vi "TagContainer-UpdateUI.vi"(7 "VIRef(Caller VI)":refnum<vi>, 8 "error in (no error)":errorcluster, 9 "force update(F)":bool, 11 "TagContainer":T1) -> (0 "error out":errorcluster, 3 "TagContainer(dup)":T1)   [LabVIEW 2017, in "TagContainer.lvlib"]
uses:
  TagContainer.lvlib
  Program Files (x86)/National Instruments/LabVIEW 2020/user.lib/_OpenG.lib/array/array.llb/Index 1D Array Elements (Variant)__ogtk.vi
  Typedef/TagContainer.ctl
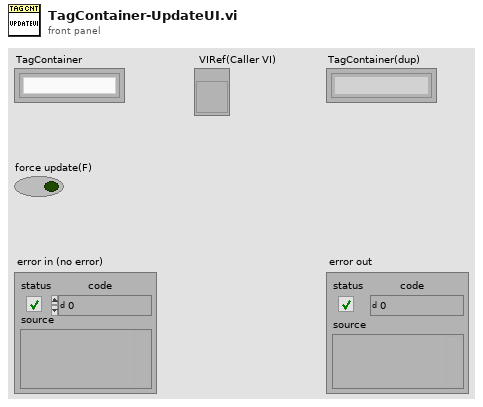
[diagram p1: front panel]
types:
  T1 = typedef "TagContainer.lvlib/TagContainer.ctl" = refnum<k1>
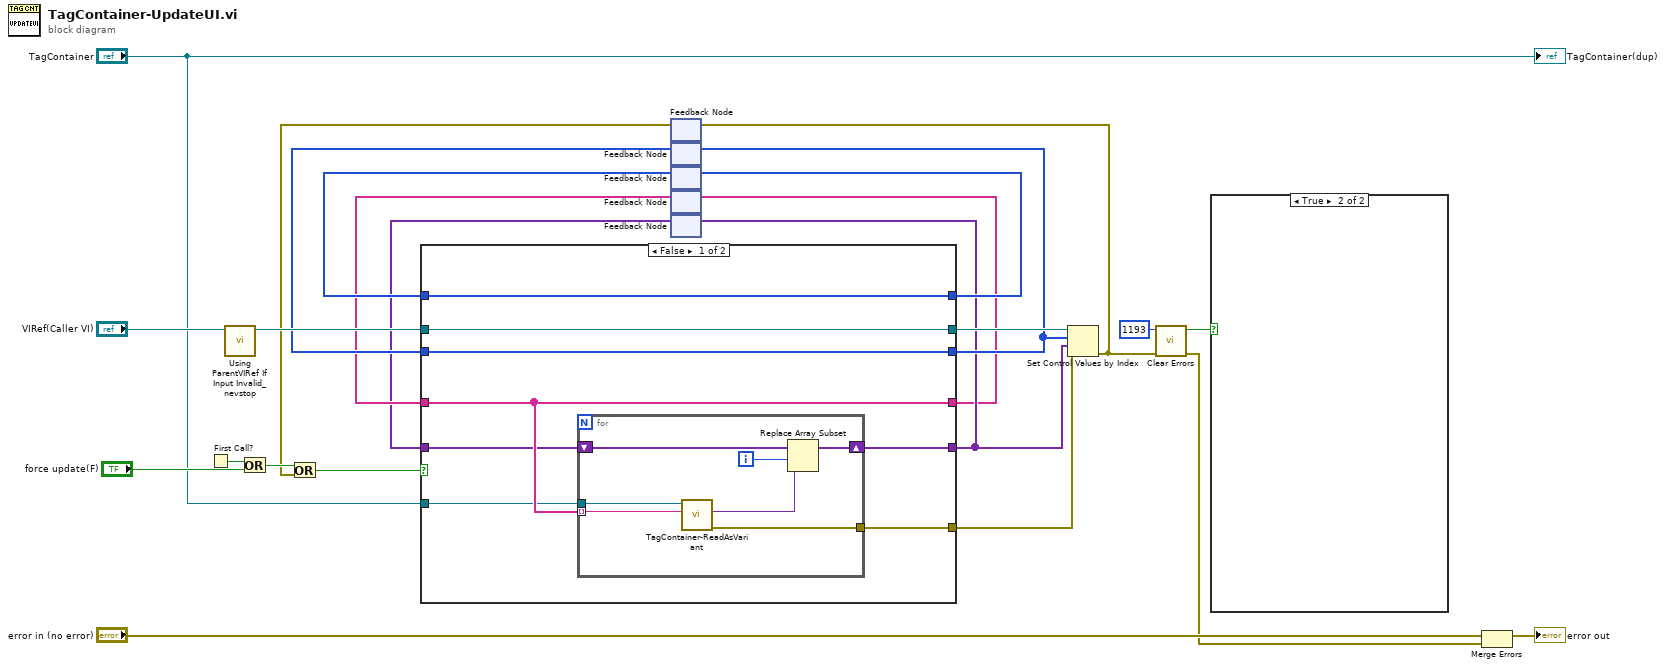
[diagram p0: block diagram]
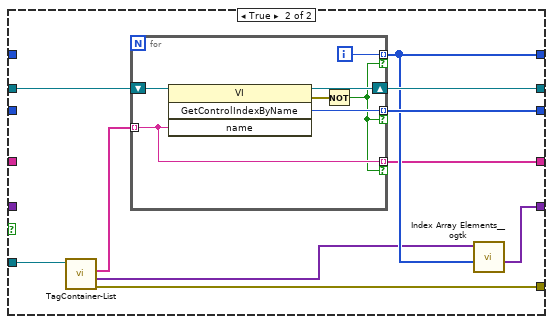
[diagram p3: hidden frame]
diagram:
  n1 = First Call?() -> (First Call?: T/F=w19:bool)
  n2 = call "Using ParentVIRef If Input Invalid_nevstop.vi"("VI Ref (calling VI)"="VIRef(Caller VI)") -> ("VI Ref"=w21:refnum<vi>)  [unwired: 5 in, 1 out]
  n3 = Or(x=w19, y="force update(F)") -> (x .or. y?=w15:bool)
  n4 = feedback #1() -> (w1:errorcluster)  [unwired: 1 in]
  n5 = Or(x=w15, y=w1) -> (x .or. y?=w3:bool)
  n6 = feedback #2() -> (w17:i32[])  [unwired: 1 in]
  n7 = feedback #3() -> (w18:i32[])  [unwired: 1 in]
  n8 = feedback #4() -> (w12:string[])  [unwired: 1 in]
  n9 = feedback #5() -> (w8:variant[])  [unwired: 1 in]
  n10 = case shown="False" w3 {
    tunnel: [w32 w49] -> w22
    tunnel: w21 -> [w32 w48]
    tunnel: [w30 w47] -> w20
    tunnel: [w31 w46] -> w16
    tunnel: w18 -> [w31 _]
    tunnel: w17 -> [w30 _]
    tunnel: [w28 w45] -> w4
    tunnel: w12 -> [w28 _]
    tunnel: [w26 w44] -> w9
    tunnel: "TagContainer" -> [w25 w43]
    tunnel: [w29 w42] -> w10
    tunnel: w8 -> [w27 _]
    frame False {
      n11 = for {
        tunnel: [w39] -> w29
        tunnel: w28 -> [w38] mode=indexing
        shift-right: [w36] -> w26
        shift-left: w27 -> [w37]
        tunnel: w25 -> [w33]
        i -> [w35]
        n12 = call "TagContainer-ReadAsVariant.vi"("name"=w38, "TagContainer"=w33) -> ("error out"=w39:errorcluster, "Value"=w34:variant)  [unwired: 5 in, 3 out]
        n13 = Replace Array Subset(array=w37, new element=w34, index=w35) -> (w36:variant[])
      }
    }
    frame True {
      n14 = call "TagContainer-List.vi"("TagContainer"=w43) -> ("error out"=w42:errorcluster, "Data"=w41:variant[], "names"=w40:string[])  [unwired: 7 in, 1 out]
      n15 = for {
        tunnel: w40 -> [w51] mode=indexing
        tunnel: [w55] -> w47 mode=indexing if=w50
        shift-right: [w56] -> w49
        shift-left: w48 -> [w53]
        tunnel: [w52] -> w46 mode=indexing if=w50
        tunnel: [w51] -> w45 mode=indexing if=w50
        i -> [w52]
        n16 = invoke class="VI" method="GetControlIndexByName"(reference=w53, "name"=w51) -> (reference out=w56:refnum<vi>, error out=w54:errorcluster, "GetControlIndexByName"=w55:i32)  [unwired: 2 in, 1 out]
        n17 = Not(x=w54) -> (.not. x?=w50:bool)
      }
      n18 = call-poly "Index Array Elements__ogtk.vi"("indices"=w46, "array"=w41) -> ("elements"=w44:variant[])  [unwired: 9 in]
    }
  }
  n19 = feedback-in #2(w20) -> ()
  n20 = feedback-in #3(w16) -> ()
  n21 = feedback-in #4(w4) -> ()
  n22 = feedback-in #5(w9) -> ()
  n23 = Set Control Values by Index(0:w22, 1:w20, 2:w9, 3:w10) -> (11:w2:errorcluster)
  n24 = feedback-in #1(w2) -> ()
  n25 = call <vilib>:"Clear Errors.vi"("error in (no error)"=w2, "specific error code to clear (0: all)"=1193) -> ("error out"=w7:errorcluster, "specific error cleared?"=w5:bool)  [unwired: 4 in]
  n26 = case shown="True" w5 {
    frame False {
    }
    frame True {
    }
  }
  n27 = Merge Errors("error in (no error)", w7) -> (→"error out":errorcluster)
  "TagContainer(dup)" <- "TagContainer"
